vi "Run Test.vi"(8 "error in (no error)":errorcluster, 10 "Words":string[](array[string]), 11 "Solver Ref":T1) -> (0 "error out":errorcluster, 1 "Valid":bool, 2 "Results":string, 3 "Avg Guesses":dbl=10.0, 5 "Min Guesses":i32, 7 "Max Guesses":i32)   [LabVIEW 2024, in "Wordle Engine.lvlib"]
uses:
  Wordle Engine.lvlib
  Scorer/Solver VI Ref Type.ctl
  Scorer/Wordle Scorer.lvlib
panel:
  out "Current Solve":i32
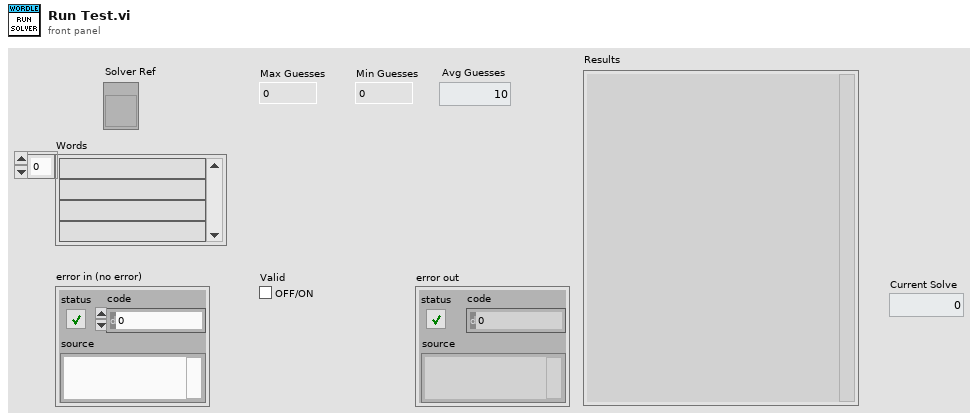
[diagram p1: front panel]
types:
  T1 = typedef "Wordle Scorer.lvlib/Solver VI Ref Type.ctl" = refnum<vi>
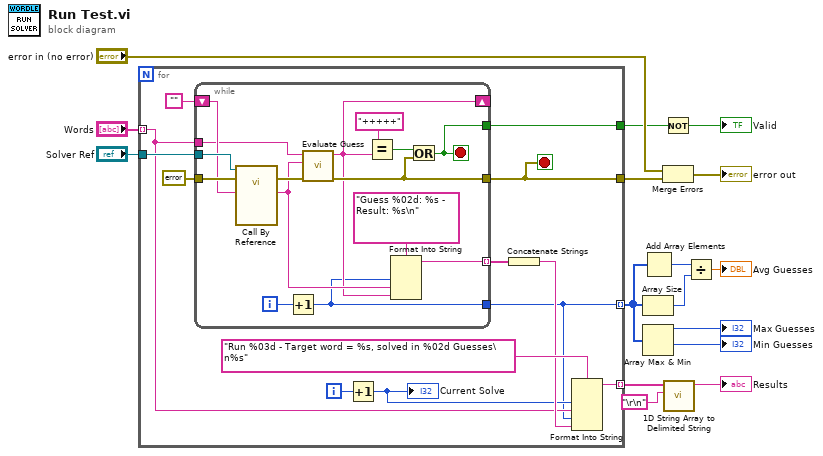
[diagram p0: block diagram]
diagram:
  n1 = for {
    tunnel: "Words" -> [w21] mode=indexing
    tunnel: "Solver Ref" -> [w29]
    tunnel: [w20] -> w9 mode=indexing
    tunnel: [w19] -> w15 mode=indexing
    tunnel: [w18] -> w6
    tunnel: [w17] -> w2
    i -> [w22]
    stop <- w18 stop-if-true
    n2 = while {
      tunnel: w29 -> [w44]
      tunnel: errorcluster {"status"=FALSE, "code"=0, "source"=""} ("error out") -> [w43]
      tunnel: [w39] -> w18
      shift-right: [w34] -> _
      shift-left: "" -> [w42]
      tunnel: w21 -> [w41]
      tunnel: [w33] -> w23 mode=indexing
      tunnel: [w31] -> w20
      tunnel: [w30] -> w17
      i -> [w32]
      stop <- w30 stop-if-true
      n3 = call-by-ref "?"(reference=w44, error in=w43, "Feedback"=w42) -> (error out=w40:errorcluster, "Guess"=w35:string)  [unwired: 10 in, 1 out]
      n4 = Increment(x=w32) -> (x+1=w31:i32)
      n5 = call "Evaluate Guess.vi"("error in"=w40, "Guess"=w35, "Current Word"=w41) -> ("error out"=w39:errorcluster, "Result"=w34:string)  [unwired: 7 in]
      n6 = Equal?(x="+++++", y=w34) -> (x = y?=w37:bool)
      n7 = Format Into String(format string="Guess %02d: %s - Result: %s\n", w31, w35, w34) -> (resulting string=w33:string)  [unwired: 2 in, 1 out]
      n8 = Or(x=w37, y=w39) -> (x .or. y?=w30:bool)
    }
    n9 = Increment(x=w22) -> (x+1=w24:i32)
    "Current Solve" <- w24
    n10 = Concatenate Strings(w23) -> (w25:string)
    n11 = Format Into String(format string="Run %03d - Target word = %s, solved in %02d Guesses\n%s", w24, w21, w20, w25) -> (resulting string=w19:string)  [unwired: 2 in, 1 out]
  }
  n12 = Array Size(array=w9) -> (size(s)=w11:i32)
  n13 = Array Max & Min(array=w9) -> (max value=→"Max Guesses":i32, min value=→"Min Guesses":i32)  [unwired: 2 out]
  n14 = Add Array Elements(numeric array=w9) -> (sum=w12:i32)
  n15 = Not(x=w2) -> (.not. x?=→"Valid":bool)
  n16 = Merge Errors("error in (no error)", w6) -> (→"error out":errorcluster)
  n17 = call <vilib>:"1D String Array to Delimited String.vi"("delimiter"="\r\n", "string array"=w15) -> ("delimited string"=→"Results":string)  [unwired: 9 in]
  n18 = Divide(x=w12, y=w11) -> (x/y=→"Avg Guesses":dbl)
